vi "Configure Volt Time Limit.vi"(8 "error in (no error)":errorcluster, 9 "Type(Up time 0)":u16(ring) items=["Up time", "Down time"], 10 "Time Value(0)":dbl min=0.0, 11 "VISA resource name":refnum<visa-resource-name>) -> (0 "error out":errorcluster, 3 "VISA resource name out":refnum<visa-resource-name>)   [LabVIEW 2020, in "IT6500.lvlib"]
doc: "This command is used to control the power supply voltage up/down time.\n\n<b>Type</b>\n0:Up time\n This command is used to control the power supply voltage rise time\n1:Down time\n This command is used to control the power supply voltage drop time"
uses:
  IT6500.lvlib
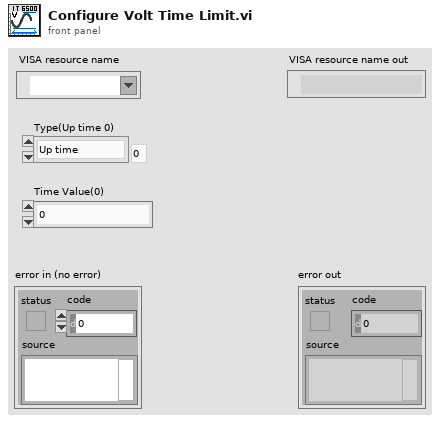
[diagram p1: front panel]
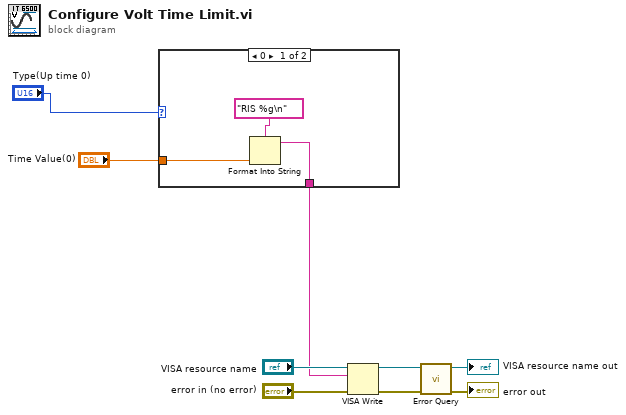
[diagram p0: block diagram]
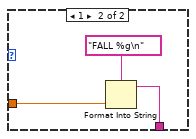
[diagram p2: hidden frame]
diagram:
  n1 = case shown="0" "Type(Up time 0)" {
    tunnel: "Time Value(0)" -> [w12 w14]
    tunnel: [w10 w13] -> w2
    frame 0 {
      n2 = Format Into String(format string="RIS %g\n", w12) -> (resulting string=w10:string)  [unwired: 2 in, 1 out]
    }
    frame 1 {
      n3 = Format Into String(format string="FALL %g\n", w14) -> (resulting string=w13:string)  [unwired: 2 in, 1 out]
    }
  }
  n4 = VISA Write(VISA resource name="VISA resource name", write buffer=w2, error in (no error)="error in (no error)") -> (VISA resource name out=w6:refnum<visa-resource-name>, error out=w7:errorcluster)  [unwired: 1 out]
  n5 = call "Error Query.vi"("error in (no error)"=w7, "VISA resource name"=w6) -> ("error out"=→"error out":errorcluster, "VISA resource name out"=→"VISA resource name out":refnum<visa-resource-name>)  [unwired: 6 in, 2 out]
